vi "Update Sparameters Ring.vi"(7 "S-par reference":refnum<vi>, 8 "error in (no error)":errorcluster, 10 "Frequencies in":dbl[](array[numeric]), 11 "S-parameters in":cdb[][](array[numeric])) -> (0 "error out":errorcluster, 1 "Number of S-parameters":i32, 2 "Frequencies out":dbl[](array[numeric]), 3 "S-parameters out":cdb[][](array[numeric]))   [LabVIEW 2023, in "NI_HFNetworkAnalysis.lvlib"]
doc: "Update a S-parameter selection ring control based on the specified S-parameters."
uses:
  NI_HFNetworkAnalysis.lvlib
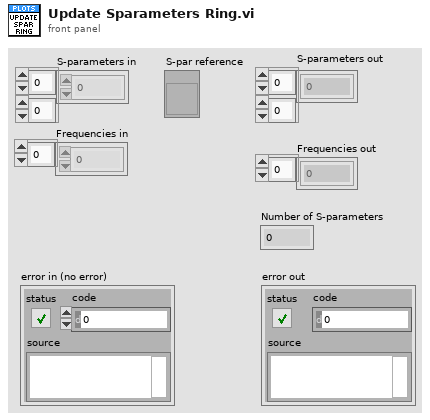
[diagram p1: front panel]
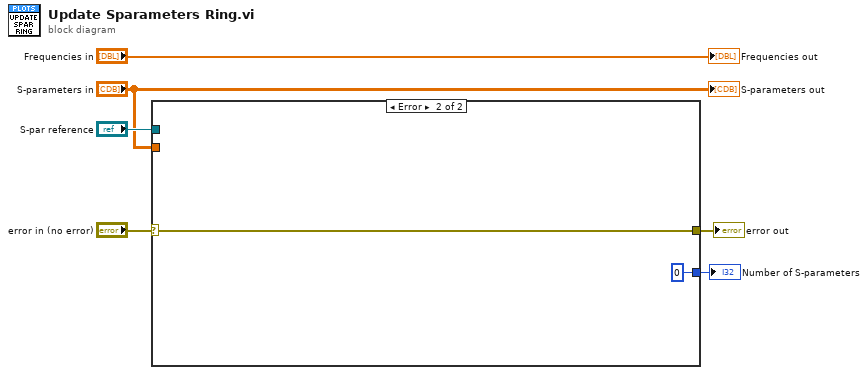
[diagram p0: block diagram]
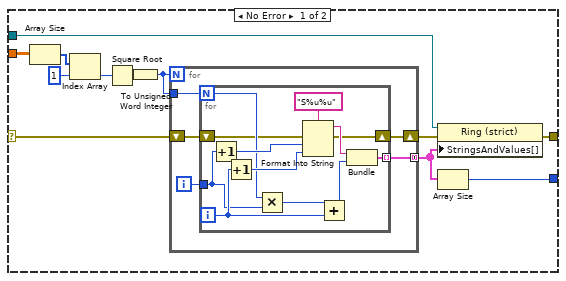
[diagram p2: hidden frame]
diagram:
  n1 = case shown="Error" "error in (no error)" {
    selector: "error in (no error)" -> [w9 w37]
    tunnel: [w18 w37] -> w6
    tunnel: "S-par reference" -> [w16 _]
    tunnel: "S-parameters in" -> [w10 _]
    tunnel: [w7 0] -> w1
    frame No Error {
      n2 = Array Size(array=w10) -> (size(s)=w11:i32[])
      n3 = Index Array(array=w11, index=1) -> (element=w13:i32)
      n4 = Square Root(x=w13) -> (sqrt(x)=w15:dbl)
      n5 = To Unsigned Word Integer(number=w15) -> (unsigned 16bit integer=w14:u16)
      n6 = for {
        N: w14 -> [_]
        tunnel: w14 -> [w23]
        tunnel: [w21] -> w8 mode=concatenating
        shift-right: [w19] -> w17
        shift-left: w9 -> [w20]
        i -> [w22]
        n7 = for {
          N: w23 -> [w26]
          tunnel: w22 -> [w27]
          tunnel: [w31] -> w21 mode=indexing
          shift-right: [w24] -> w19
          shift-left: w20 -> [w25]
          i -> [w34]
          n8 = Increment(x=w27) -> (x+1=w29:i32)
          n9 = Increment(x=w34) -> (x+1=w30:i32)
          n10 = Multiply(x=w26, y=w27) -> (x*y=w28:i32)
          n11 = Format Into String(format string="S%u%u", error in=w25, w29, w30) -> (resulting string=w33:string, error out=w24:errorcluster)  [unwired: 1 in]
          n12 = Add(x=w28, y=w34) -> (x+y=w32:i32)
          n13 = Bundle(w33, w32) -> (w31:cluster{string, i32})  [unwired: 1 in]
        }
      }
      n14 = property on="Property Node" class="Ring (strict)"(reference=w16, error in=w17, "StringsAndValues[]"=w8) -> (error out=w18:errorcluster)  [unwired: 1 out]
      n15 = Array Size(array=w8) -> (size(s)=w7:i32)
    }
    frame Error {
    }
  }
  "error out" <- w6
  "Number of S-parameters" <- w1
  "S-parameters out" <- "S-parameters in"
  "Frequencies out" <- "Frequencies in"
